vi "Global_CMD.vi"() -> ()   [LabVIEW 2017, in "SRX SubSystem.lvlib"]
uses:
  SRX SubSystem.lvlib
  _SHARE ALL/RoboRio Share All/SRX Share All/TypeDefs SRX/Cluster_SRX_Mode and Value.ctl
  System Drivers/Phoenix-LabVIEW/Motor Controller/Controls/CTRE_Phoenix_MotorControl_ControlMode.ctl
panel:
  in  "CMD_SRX Arm_ Mode":T1 {"Mode" items=["PercentOutput"=0, "Position"=1, "Velocity"=2, "Current"=3, "Follower"=5, "MotionProfile"=6, "MotionMagic"=7, "MotionMagicArc"=8, "MotionProfileArc"=10, "Disabled"=15]}
  # "The Names of the Data items in the Global Variable MUST describe who the Single Writer is\nNaming Convention for Command Globals is:   \n\nCMD_SubSystem_Data Name\nExample:\nCMD_Drive_Mode\nCMD_Hopper_Fire Ball"
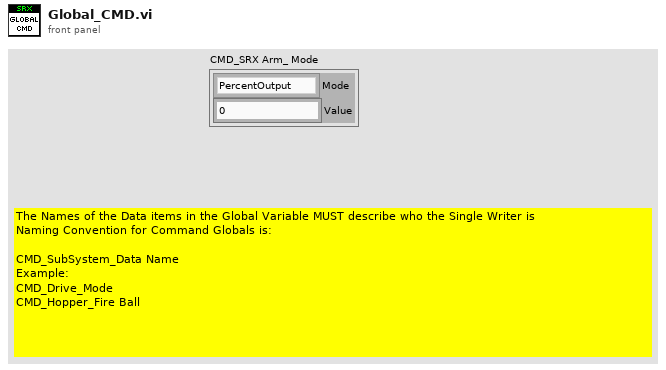
[diagram p1: front panel]
types:
  T1 = typedef "Cluster_SRX_Mode and Value.ctl" = cluster{"Mode":T2, "Value":dbl}
  T2 = typedef "CTRE_Phoenix_MotorControl_ControlMode.ctl" = u16
diagram:
